vi "loadFile.vi"(7 "LabVIEW Web Service Request":refnum<class "Web Request.lvclass">, 11 "fn":string) -> ()   [LabVIEW 2014]
uses:
  <vilib>/wsapi/Web Request.lvclass
  Audio/Controls/playback state.ctl
  Controls/Application Data.vi
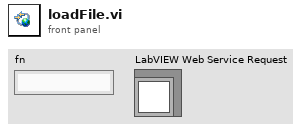
[diagram p1: front panel]
types:
  T1 = typedef "playback state.ctl" = enum16{"Load File", "Save File", "Play", "Record", "Stop", "Rewind"}
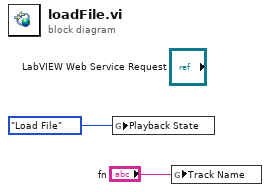
[diagram p0: block diagram]
diagram:
  n1 = global write "Application Data.vi" "Playback State"(playback_state."Load File" ("Playback State")) -> ()
  n2 = global write "Application Data.vi" "Track Name"("fn") -> ()
